vi "Add Path.vi"(0 "Origin":cdb, 1 "Move":T3, 2 "To Location":cdb, 4 "Paths in":T1) -> (7 "Paths out":T1)   [LabVIEW 2020, in "AoC 2022.lvlib"]
uses:
  AoC 2022.lvlib
  Paths.ctl
  <vilib>/Utility/miscctls.llb/LVMapReplaceAction.ctl
  Direction.ctl
  Path.ctl
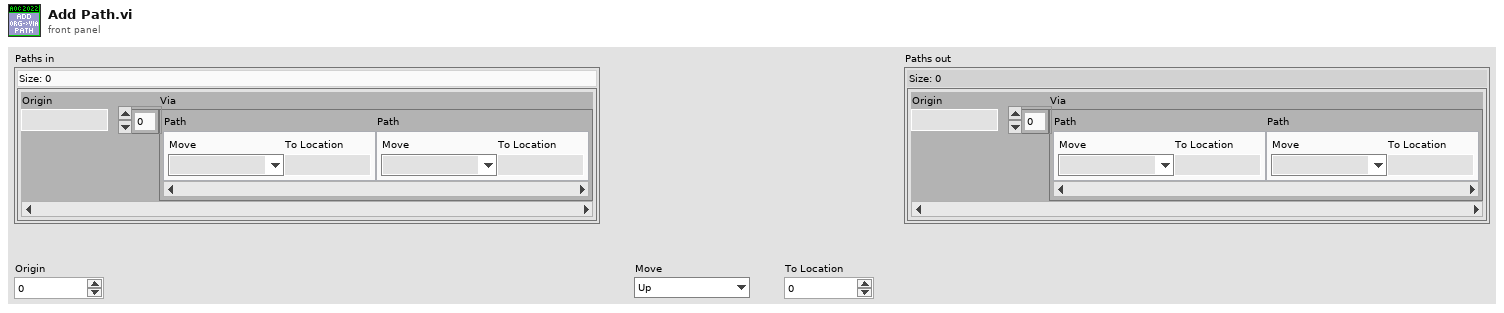
[diagram p1: front panel]
types:
  T1 = typedef "AoC 2022.lvlib/Paths.ctl" = map{cdb, T2[]}
  T2 = typedef "AoC 2022.lvlib/Path.ctl" = cluster{"Move":T3, "To Location":cdb}
  T3 = typedef "AoC 2022.lvlib/Direction.ctl" = enum16{"Up", "UpRight", "Right", "DownRight", "Down", "DownLeft", "Left", "UpLeft", "Stay"}
  T4 = typedef "LVMapReplaceAction.ctl" = enum32{"Modify Entry only if found", "Add or Modify Entry", "Delete Entry"}
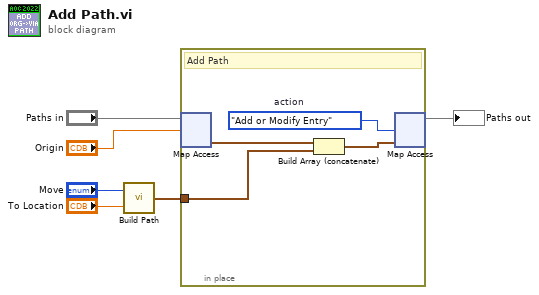
[diagram p0: block diagram]
diagram:
  n1 = call "Build Path.vi"("To Location"="To Location", "Move"="Move") -> ("Path"=w1:T2)
  n2 = in-place {
    in-place-border: w1 -> [w7]
    w8 = LVMapReplaceAction."Add or Modify Entry"  # action
    # "Add Path"
    n3 = in-place-map #1("Paths in", "Origin") -> (w10:T2[])  [unwired: 1 in, 1 out]
    n4 = Build Array (concatenate)(w10, w7) -> (w9:T2[])
    n5 = in-place-map #1(w9, w8) -> (→"Paths out":T1)  [unwired: 2 out]
  }
